vi "RWRHandling.vi"(0 "VISA in":refnum<visa-resource-name>, 1 "Dictionary":refnum<vi>, 2 "H2F Frame":refnum<vi>, 3 "Recieved Data":T1, 4 "RWR?":bool, 5 "error in (no error)":errorcluster, 6 "SensorArr Ref":refnum<vi>, 7 "On/Off Data Ref":refnum<vi>, 8 "Read Data":refnum<vi>, 9 "SendCmdLED":refnum<vi>, 11 "RecCmdLED":refnum<vi>) -> (14 "VISA Refnum out":refnum<visa-resource-name>, 15 "Recieved Data Out":T1, 16 "UART written count":u32, 19 "error out":errorcluster)   [LabVIEW 2018]
uses:
  TypeDefs/recDataClust.ctl
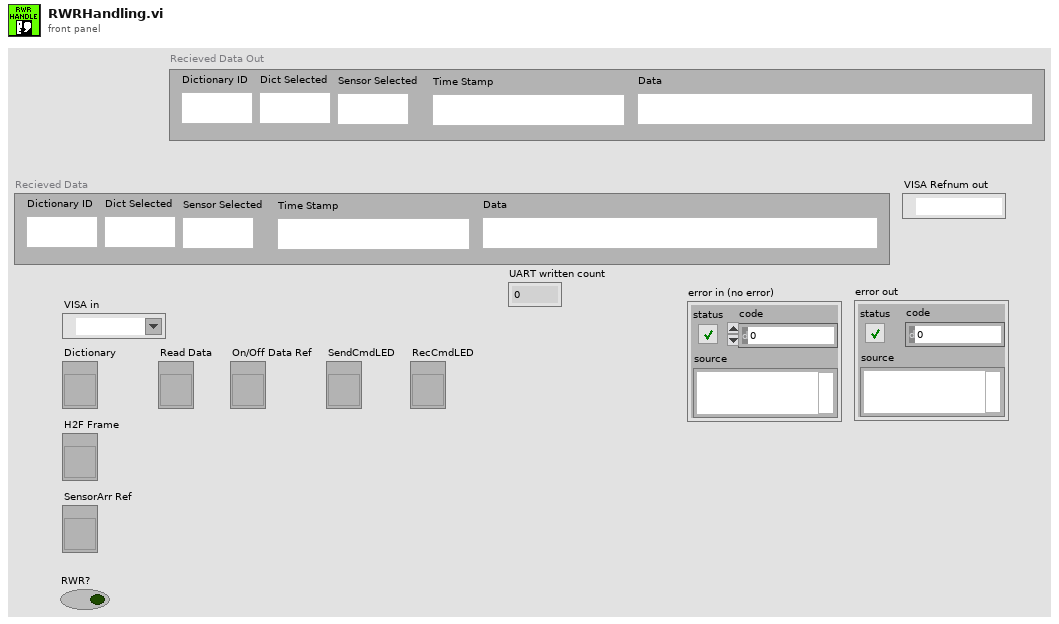
[diagram p1: front panel]
types:
  T1 = typedef "recDataClust.ctl" = cluster{"Dictionary ID":string, "Dict Selected":string, "Sensor Selected":string, "Time Stamp":string, "Data":string}
  T2 = enum32{"No Selection", "WRITE", "READ", "WRITE -> READ", "READ -> WRITE -> READ", "ON/OFF", "NO ARGS"}
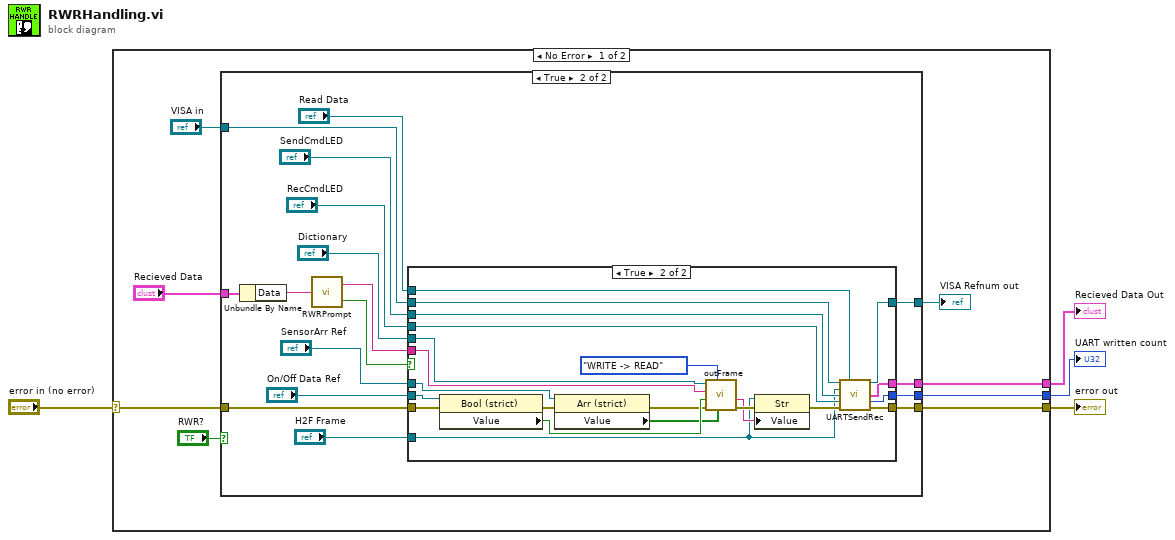
[diagram p0: block diagram]
diagram:
  n1 = case shown="No Error" "error in (no error)" {
    selector: "error in (no error)" -> [w11 w56]
    tunnel: [w12 w56] -> w3
    tunnel: [w6 _] -> w2
    tunnel: [w5 _] -> w1
    frame No Error {
      n2 = case shown="True" "RWR?" {
        tunnel: w11 -> [w14 w28]
        tunnel: [w14 w26] -> w12
        tunnel: "VISA in" -> [w13 w25]
        tunnel: "Recieved Data" -> [_ w27]
        tunnel: [w13 w24] -> w7
        tunnel: [_ w16] -> w5
        tunnel: [_ w15] -> w6
        frame False {
        }
        frame True {
          n3 = Unbundle By Name(w27) -> ("Data"=w31:string)
          n4 = call "RWRPrompt.vi"("Value Present in Detector 2"=w31) -> ("Value to update in Detector 2"=w29:string, "Cancel Pressed"=w30:bool)
          n5 = case shown="True" w30 {
            tunnel: w29 -> [_ w55]
            tunnel: w28 -> [w33 w51]
            tunnel: [w33 w49] -> w26
            tunnel: w25 -> [w32 w44]
            tunnel: [w32 w43] -> w24
            tunnel: "SensorArr Ref" -> [_ w42]
            tunnel: "Dictionary" -> [_ w41]
            tunnel: "Read Data" -> [_ w34]
            tunnel: "RecCmdLED" -> [_ w40]
            tunnel: "SendCmdLED" -> [_ w39]
            tunnel: "On/Off Data Ref" -> [_ w38]
            tunnel: "H2F Frame" -> [_ w37]
            tunnel: [_ w36] -> w16
            tunnel: [_ w35] -> w15
            frame False {
            }
            frame True {
              n6 = property on="Property Node" class="Bool (strict)"(reference=w38, error in=w51) -> (error out=w52:errorcluster, "Value"=w54:bool)  [unwired: 1 out]
              n7 = property on="Property Node" class="Arr (strict)"(reference=w42, error in=w52) -> (error out=w46:errorcluster, "Value"=w53:bool[])  [unwired: 1 out]
              n8 = call "outFrame.vi"("Sensor Array"=w53, "Select Macro Function"=T2."WRITE -> READ", "error in (no error)"=w46, "On/Off Data"=w54, "Write Data (HEX)"=w55, "Cluster in"=w41) -> ("error out"=w48:errorcluster, "H2F Frame"=w47:string)  [unwired: 4 in]
              n9 = property on="Property Node" class="Str"(reference=w37, error in=w48, "Value"=w47) -> (error out=w45:errorcluster)  [unwired: 1 out]
              n10 = call "UARTSendRec.vi"("VISA resource name in"=w44, "Read Data Ref"=w34, "H2F Frame Ref"=w37, "Send LED Ref"=w39, "Rec LED Ref"=w40, "error in (no error)"=w45) -> ("VISA resource name out"=w43:refnum<visa-resource-name>, "Recieved Data"=w36:T1, "UART written count"=w35:u32, "error out"=w49:errorcluster)  [unwired: 6 in]
            }
          }
        }
      }
      "VISA Refnum out" <- w7
    }
    frame Error {
    }
  }
  "error out" <- w3
  "UART written count" <- w2
  "Recieved Data Out" <- w1
